vi "Process Effect Messages.vi"(8 "error in (no error)":errorcluster, 11 "Effect Unit in":refnum<class "Effect Unit.lvclass">) -> (0 "error out":errorcluster, 3 "Effect Unit out":refnum<class "Effect Unit.lvclass">)   [LabVIEW 2019, in "Effect Unit.lvclass"]
uses:
  Effect Unit.lvclass
  Effect Unit.lvclass/Effect Unit.ctl
  Packed Libraries/Messaging.lvlibp
  Packed Libraries/Audio Processing.lvlibp
  Plugin Interfaces/Effect Interface/Effect Interface.lvlibp/Effect Interface Class/Effect Interface.lvclass
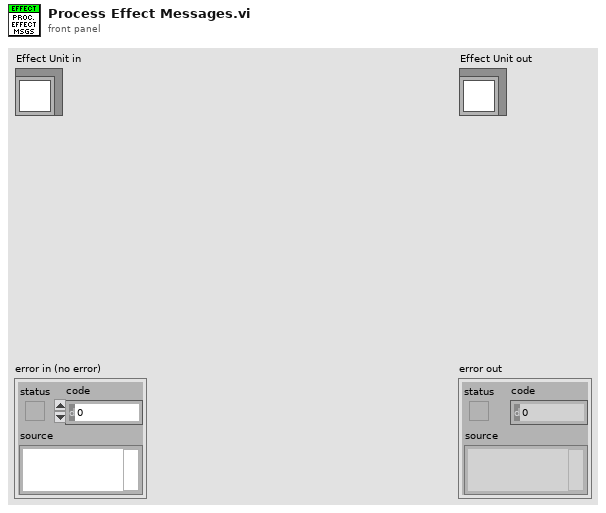
[diagram p1: front panel]
types:
  T1 = typedef "Effect Unit.lvclass/Effect Info.ctl" = cluster{"ID":string, "Message Queue":refnum<queue>, "Effect Interface":refnum<class "Effect Interface.lvclass">}
  T2 = typedef "Messaging.lvlib/Message Cluster.ctl" = cluster{"Event":string, "Source":string, "Target":string, "Data":variant}
  T3 = typedef "Audio Processing.lvlibp/Value Cluster.ctl" = cluster{"Value":dbl, "Properties":T4}
  T4 = typedef "Audio Processing.lvlibp/Value Properties.ctl" = cluster{"Lower":dbl, "Upper":dbl, "Default":dbl, "Increment":dbl}
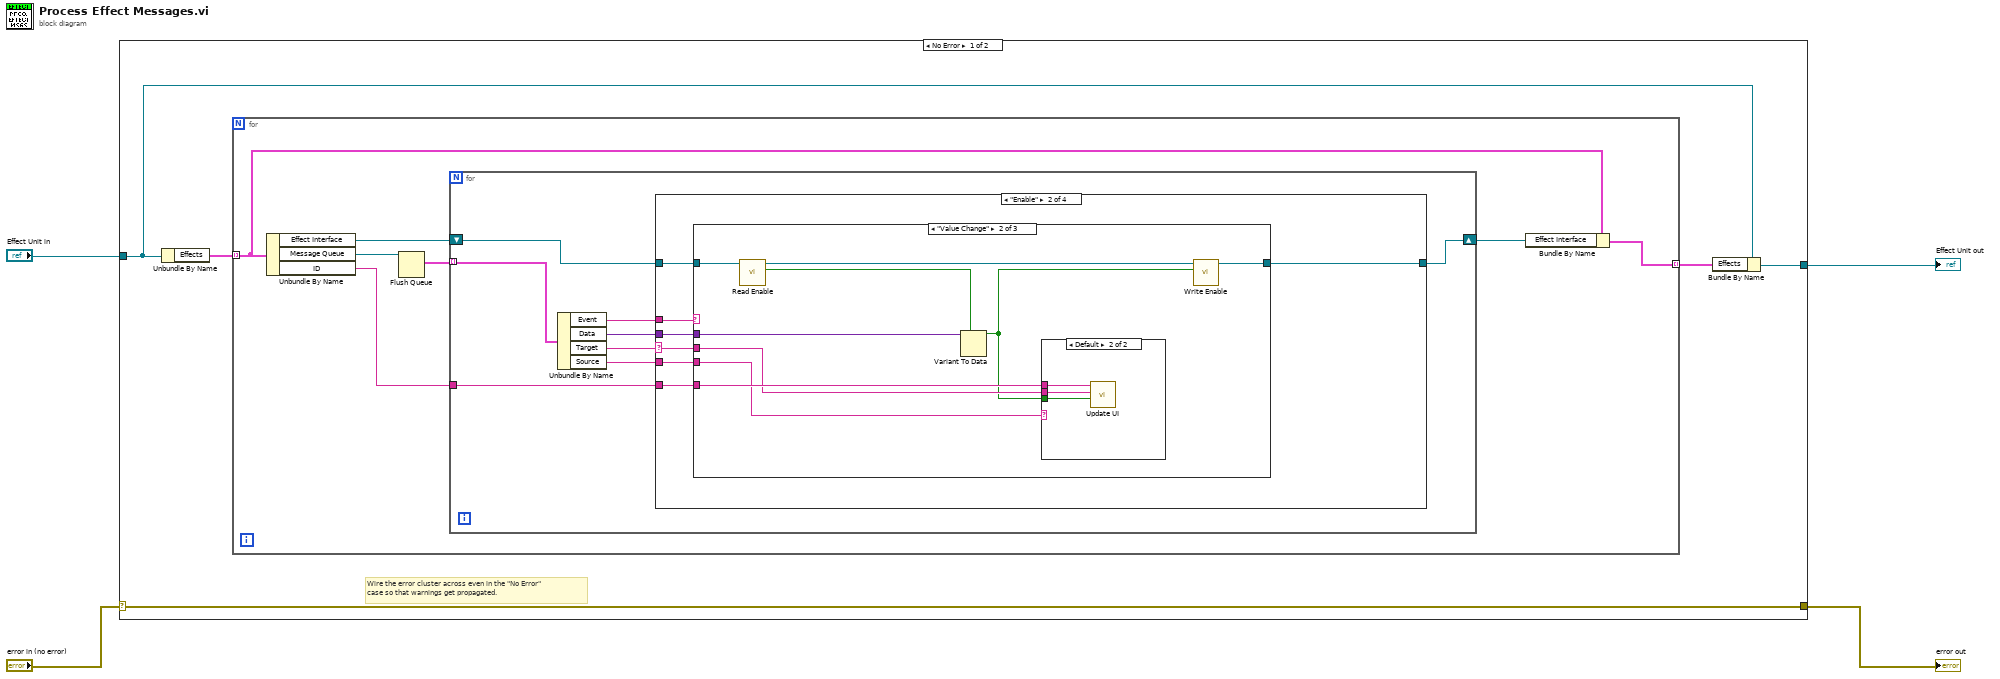
[diagram p0: block diagram]
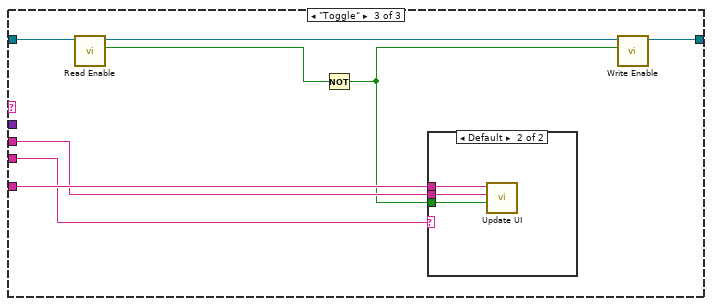
[diagram p5: hidden frame]
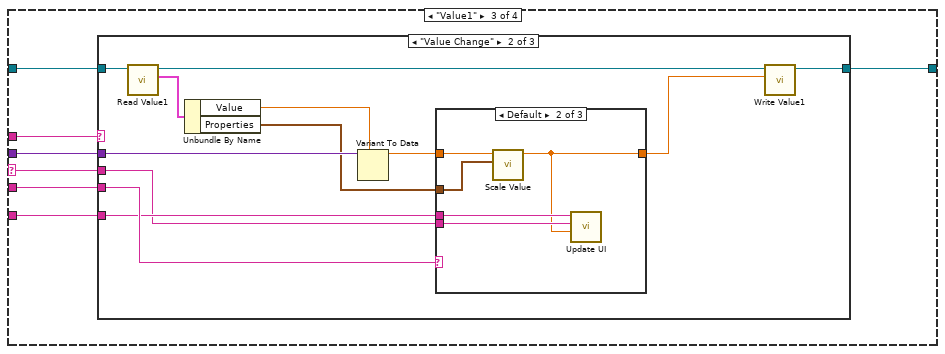
[diagram p7: hidden frame]
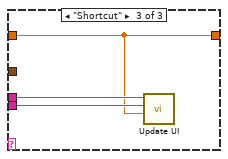
[diagram p10: hidden frame]
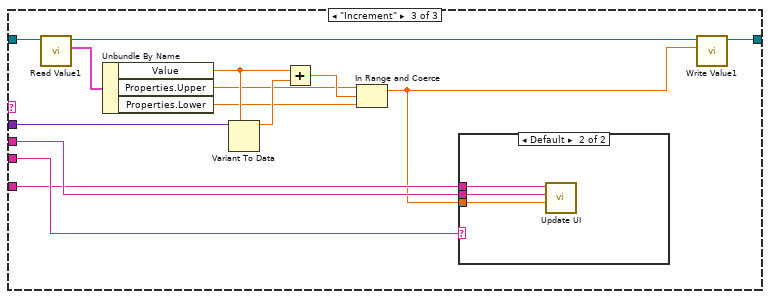
[diagram p11: hidden frame]
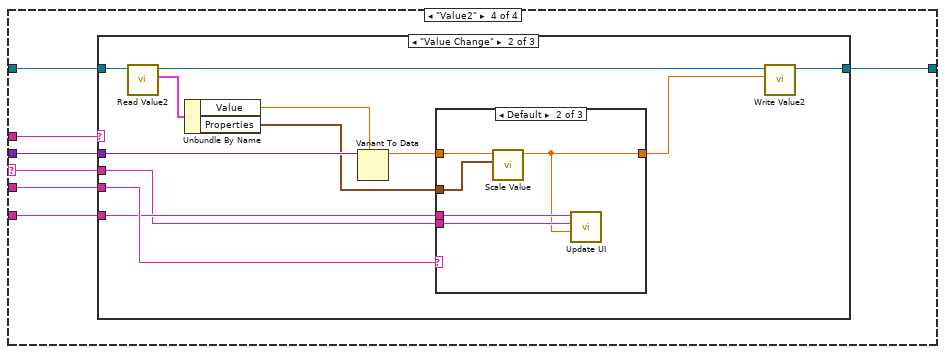
[diagram p13: hidden frame]
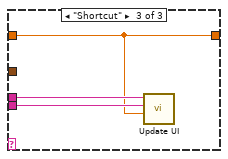
[diagram p16: hidden frame]
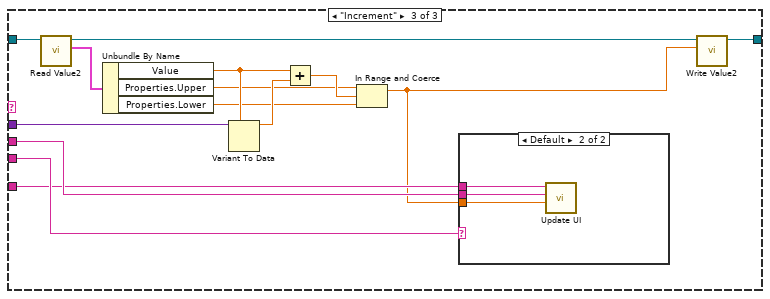
[diagram p17: hidden frame]
diagram:
  n1 = case shown="No Error" "error in (no error)" {
    selector: "error in (no error)" -> [w9 w150]
    tunnel: [w9 w150] -> w1
    tunnel: [w7 w149] -> w2
    tunnel: "Effect Unit in" -> [w6 w149]
    frame No Error {
      # "Wire the error cluster across even in the \"No Error\"\ncase so that warnings get propagated."
      n2 = Unbundle By Name(w6) -> ("Effects"=w5:T1[])
      n3 = for {
        tunnel: [w11] -> w8 mode=indexing
        tunnel: w5 -> [w10] mode=indexing
        n4 = Unbundle By Name(w10) -> ("Effect Interface"=w13:refnum<class "Effect Interface.lvclass">, "Message Queue"=w16:refnum<queue>, "ID"=w14:string)
        n5 = Flush Queue(queue=w16) -> (remaining elements=w15:T2[])  [unwired: 1 in, 2 out]
        n6 = for {
          shift-right: [w21] -> w12
          shift-left: w13 -> [w22]
          tunnel: w15 -> [w24] mode=indexing
          tunnel: w14 -> [w17]
          n7 = Unbundle By Name(w24) -> ("Event"=w20:string, "Data"=w19:variant, "Target"=w23:string, "Source"=w18:string)
          n8 = case shown="\"Enable\"" w23 {
            selector: w23 -> [_ w27 w59 w105]
            tunnel: w22 -> [w25 w31 w63 w109]
            tunnel: [w25 w29 w62 w108] -> w21
            tunnel: w20 -> [_ w32 w61 w107]
            tunnel: w19 -> [_ w30 w60 w106]
            tunnel: w18 -> [_ w28 w57 w103]
            tunnel: w17 -> [_ w26 w58 w104]
            frame Default {
            }
            frame "Enable" {
              n9 = case shown="\"Value Change\"" w32 {
                tunnel: w31 -> [w33 w35 w49]
                tunnel: w30 -> [_ w42 _]
                tunnel: [w33 w37 w47] -> w29
                tunnel: w28 -> [_ w39 w51]
                tunnel: w27 -> [_ w40 w52]
                tunnel: w26 -> [_ w41 w53]
                frame Default {
                }
                frame "Value Change" {
                  n10 = call "Read Enable.vi"("Effect Interface in"=w35) -> ("Enable"=w34:bool, "Effect Interface out"=w36:refnum<class "Effect Interface.lvclass">)  [unwired: 9 in]
                  n11 = Variant To Data(type=w34, Variant=w42) -> (data=w38:bool)  [unwired: 1 in, 1 out]
                  n12 = case shown="Default" w39 {
                    tunnel: w41 -> [_ w45]
                    tunnel: w40 -> [_ w44]
                    tunnel: w38 -> [_ w43]
                    frame "UI" {
                    }
                    frame Default {
                      n13 = call "Update UI.vi"("Data"=w43, "Target"=w44, "ID"=w45) -> ()  [unwired: 8 in, 1 out]
                    }
                  }
                  n14 = call "Write Enable.vi"("Enable"=w38, "Effect Interface in"=w36) -> ("Effect Interface out"=w37:refnum<class "Effect Interface.lvclass">)  [unwired: 9 in]
                }
                frame "Toggle" {
                  n15 = call "Read Enable.vi"("Effect Interface in"=w49) -> ("Enable"=w50:bool, "Effect Interface out"=w48:refnum<class "Effect Interface.lvclass">)  [unwired: 9 in]
                  n16 = Not(x=w50) -> (.not. x?=w46:bool)
                  n17 = case shown="Default" w51 {
                    tunnel: w53 -> [_ w56]
                    tunnel: w52 -> [_ w55]
                    tunnel: w46 -> [_ w54]
                    frame "UI" {
                    }
                    frame Default {
                      n18 = call "Update UI.vi"("Data"=w54, "Target"=w55, "ID"=w56) -> ()  [unwired: 8 in, 1 out]
                    }
                  }
                  n19 = call "Write Enable.vi"("Enable"=w46, "Effect Interface in"=w48) -> ("Effect Interface out"=w47:refnum<class "Effect Interface.lvclass">)  [unwired: 9 in]
                }
              }
            }
            frame "Value1" {
              n20 = case shown="\"Value Change\"" w61 {
                tunnel: [w64 w66 w87] -> w62
                tunnel: w63 -> [w64 w69 w89]
                tunnel: w60 -> [_ w75 w99]
                tunnel: w57 -> [_ w73 w98]
                tunnel: w59 -> [_ w71 w97]
                tunnel: w58 -> [_ w72 w96]
                frame Default {
                }
                frame "Value Change" {
                  n21 = call "Read Value1.vi"("Effect Interface in"=w69) -> ("Value Cluster"=w68:T3, "Effect Interface out"=w67:refnum<class "Effect Interface.lvclass">)  [unwired: 9 in]
                  n22 = Unbundle By Name(w68) -> ("Value"=w76:dbl, "Properties"=w70:T4)
                  n23 = Variant To Data(type=w76, Variant=w75) -> (data=w74:dbl)  [unwired: 1 in, 1 out]
                  n24 = case shown="Default" w73 {
                    tunnel: w74 -> [w77 w80 w83]
                    tunnel: w71 -> [_ w82 w85]
                    tunnel: w72 -> [_ w81 w84]
                    tunnel: [w77 w78 w83] -> w65
                    tunnel: w70 -> [_ w79 _]
                    frame "UI" {
                    }
                    frame Default {
                      n25 = call "Scale Value.vi"("Properties"=w79, "Value"=w80) -> ("Scaled Value"=w78:dbl)  [unwired: 9 in]
                      n26 = call "Update UI.vi"("Data"=w78, "Target"=w82, "ID"=w81) -> ()  [unwired: 8 in, 1 out]
                    }
                    frame "Shortcut" {
                      n27 = call "Update UI.vi"("Data"=w83, "Target"=w85, "ID"=w84) -> ()  [unwired: 8 in, 1 out]
                    }
                  }
                  n28 = call "Write Value1.vi"("Value1"=w65, "Effect Interface in"=w67) -> ("Effect Interface out"=w66:refnum<class "Effect Interface.lvclass">)  [unwired: 9 in]
                }
                frame "Increment" {
                  n29 = call "Read Value1.vi"("Effect Interface in"=w89) -> ("Value Cluster"=w90:T3, "Effect Interface out"=w88:refnum<class "Effect Interface.lvclass">)  [unwired: 9 in]
                  n30 = Unbundle By Name(w90) -> ("Value"=w95:dbl, "Properties.Upper"=w92:dbl, "Properties.Lower"=w91:dbl)
                  n31 = Variant To Data(type=w95, Variant=w99) -> (data=w94:dbl)  [unwired: 1 in, 1 out]
                  n32 = Add(x=w95, y=w94) -> (x+y=w93:dbl)
                  n33 = In Range and Coerce(upper limit=w92, x=w93, lower limit=w91) -> (coerced(x)=w86:dbl)  [unwired: 1 out]
                  n34 = case shown="Default" w98 {
                    tunnel: w86 -> [_ w102]
                    tunnel: w97 -> [_ w101]
                    tunnel: w96 -> [_ w100]
                    frame "UI" {
                    }
                    frame Default {
                      n35 = call "Update UI.vi"("Data"=w102, "Target"=w101, "ID"=w100) -> ()  [unwired: 8 in, 1 out]
                    }
                  }
                  n36 = call "Write Value1.vi"("Value1"=w86, "Effect Interface in"=w88) -> ("Effect Interface out"=w87:refnum<class "Effect Interface.lvclass">)  [unwired: 9 in]
                }
              }
            }
            frame "Value2" {
              n37 = case shown="\"Value Change\"" w107 {
                tunnel: [w110 w112 w133] -> w108
                tunnel: w109 -> [w110 w115 w135]
                tunnel: w106 -> [_ w121 w145]
                tunnel: w103 -> [_ w119 w144]
                tunnel: w105 -> [_ w117 w143]
                tunnel: w104 -> [_ w118 w142]
                frame Default {
                }
                frame "Value Change" {
                  n38 = call "Read Value2.vi"("Effect Interface in"=w115) -> ("Value Cluster"=w114:T3, "Effect Interface out"=w113:refnum<class "Effect Interface.lvclass">)  [unwired: 9 in]
                  n39 = Unbundle By Name(w114) -> ("Value"=w122:dbl, "Properties"=w116:T4)
                  n40 = Variant To Data(type=w122, Variant=w121) -> (data=w120:dbl)  [unwired: 1 in, 1 out]
                  n41 = case shown="Default" w119 {
                    tunnel: w120 -> [w123 w126 w129]
                    tunnel: w117 -> [_ w128 w131]
                    tunnel: w118 -> [_ w127 w130]
                    tunnel: [w123 w124 w129] -> w111
                    tunnel: w116 -> [_ w125 _]
                    frame "UI" {
                    }
                    frame Default {
                      n42 = call "Scale Value.vi"("Properties"=w125, "Value"=w126) -> ("Scaled Value"=w124:dbl)  [unwired: 9 in]
                      n43 = call "Update UI.vi"("Data"=w124, "Target"=w128, "ID"=w127) -> ()  [unwired: 8 in, 1 out]
                    }
                    frame "Shortcut" {
                      n44 = call "Update UI.vi"("Data"=w129, "Target"=w131, "ID"=w130) -> ()  [unwired: 8 in, 1 out]
                    }
                  }
                  n45 = call "Write Value2.vi"("Value2"=w111, "Effect Interface in"=w113) -> ("Effect Interface out"=w112:refnum<class "Effect Interface.lvclass">)  [unwired: 9 in]
                }
                frame "Increment" {
                  n46 = call "Read Value2.vi"("Effect Interface in"=w135) -> ("Value Cluster"=w136:T3, "Effect Interface out"=w134:refnum<class "Effect Interface.lvclass">)  [unwired: 9 in]
                  n47 = Unbundle By Name(w136) -> ("Value"=w141:dbl, "Properties.Upper"=w138:dbl, "Properties.Lower"=w137:dbl)
                  n48 = Variant To Data(type=w141, Variant=w145) -> (data=w140:dbl)  [unwired: 1 in, 1 out]
                  n49 = Add(x=w141, y=w140) -> (x+y=w139:dbl)
                  n50 = In Range and Coerce(upper limit=w138, x=w139, lower limit=w137) -> (coerced(x)=w132:dbl)  [unwired: 1 out]
                  n51 = case shown="Default" w144 {
                    tunnel: w132 -> [_ w148]
                    tunnel: w143 -> [_ w147]
                    tunnel: w142 -> [_ w146]
                    frame "UI" {
                    }
                    frame Default {
                      n52 = call "Update UI.vi"("Data"=w148, "Target"=w147, "ID"=w146) -> ()  [unwired: 8 in, 1 out]
                    }
                  }
                  n53 = call "Write Value2.vi"("Value2"=w132, "Effect Interface in"=w134) -> ("Effect Interface out"=w133:refnum<class "Effect Interface.lvclass">)  [unwired: 9 in]
                }
              }
            }
          }
        }
        n54 = Bundle By Name(cluster=w10, "Effect Interface"=w12) -> (w11:T1)
      }
      n55 = Bundle By Name(cluster=w6, "Effects"=w8) -> (w7:refnum<class "Effect Unit.lvclass">)
    }
    frame Error {
    }
  }
  "error out" <- w1
  "Effect Unit out" <- w2
